vi "finishPulses.vi"(8 "error in (no error)":errorcluster, 11 "ScriptEvent in":refnum<class "ScriptEvent.lvclass">) -> (0 "error out":errorcluster, 2 "pulse finish":refnum<class "ScriptEvent.lvclass">, 3 "ScriptEvent out":refnum<class "ScriptEvent.lvclass">)   [LabVIEW 2011, in "Tools.lvlib" / "Scripting.lvlib" / "ScriptEvent.lvclass"]
uses:
  ScriptEvent.lvclass
  DatabaseHelpers/Database Objects/Channel/DigitalChannel/DigitalChannel.lvclass
  ScriptEvent.lvclass/ScriptEvent.ctl
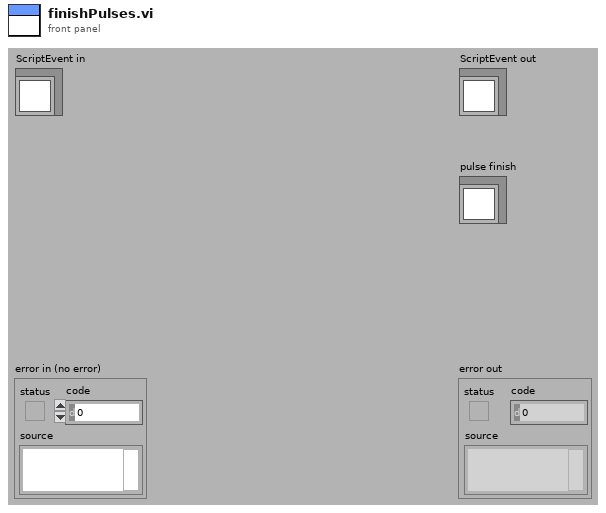
[diagram p1: front panel]
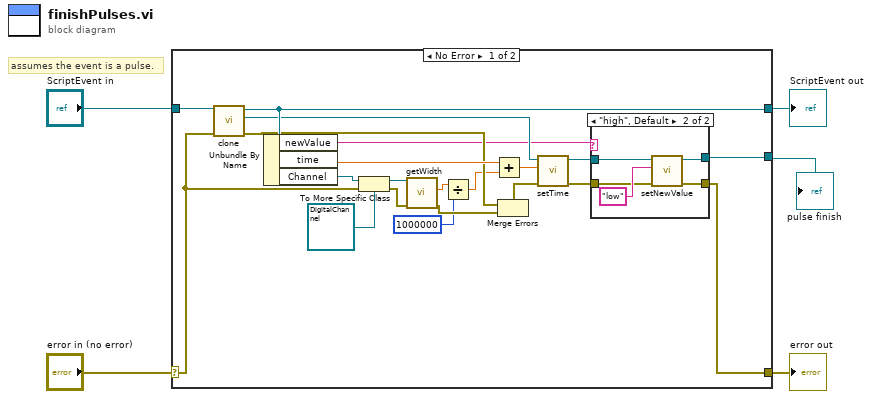
[diagram p0: block diagram]
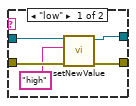
[diagram p2: hidden frame]
diagram:
  # "assumes the event is a pulse."
  n1 = case shown="No Error" "error in (no error)" {
    selector: "error in (no error)" -> [w21 w38]
    tunnel: [w10 w38] -> w4
    tunnel: [w25 w37] -> w2
    tunnel: "ScriptEvent in" -> [w26 w37]
    tunnel: [w9 _] -> w1
    frame No Error {
      n2 = call-dynamic "clone.vi"("error in (no error)"=w21, "ScriptEvent in"=w26) -> ("error out"=w18:errorcluster, "clone"=w20:refnum<class "ScriptEvent.lvclass">, "ScriptEvent out"=w25:refnum<class "ScriptEvent.lvclass">)  [unwired: 7 in]
      n3 = Unbundle By Name(w25) -> ("newValue"=w13:string, "time"=w24:dbl, "Channel"=w23:refnum<class "Channel.lvclass">)
      n4 = To More Specific Class(target class=refnum<class "DigitalChannel.lvclass"> refnum ("Tools.lvlib:DatabaseHelpers.lvlib:DigitalChannel.lvclass"), reference=w23, error in=w21) -> (specific class reference=w16:refnum<class "DigitalChannel.lvclass">, error out=w15:errorcluster)
      n5 = call "getWidth.vi"("error in (no error)"=w15, "DigitalChannel.lvclass in"=w16) -> ("error out"=w14:errorcluster, "width"=w8:dbl)  [unwired: 7 in, 1 out]
      n6 = Divide(x=w8, y=1000000) -> (x/y=w7:dbl)
      n7 = Add(x=w24, y=w7) -> (x+y=w19:dbl)
      n8 = Merge Errors(w18, w14) -> (w17:errorcluster)
      n9 = call "setTime.vi"("error in (no error)"=w17, "time"=w19, "ScriptEvent.lvclass in"=w20) -> ("error out"=w11:errorcluster, "ScriptEvent.lvclass out"=w12:refnum<class "ScriptEvent.lvclass">)  [unwired: 7 in]
      n10 = case shown="\"high\", Default" w13 {
        tunnel: w12 -> [w31 w36]
        tunnel: w11 -> [w30 w34]
        tunnel: [w29 w33] -> w10
        tunnel: [w28 w32] -> w9
        frame "low" {
          n11 = call "setNewValue.vi"("error in (no error)"=w30, "newValue"="high", "ScriptEvent.lvclass in"=w31) -> ("error out"=w29:errorcluster, "ScriptEvent.lvclass out"=w28:refnum<class "ScriptEvent.lvclass">)  [unwired: 7 in]
        }
        frame "high", Default {
          n12 = call "setNewValue.vi"("error in (no error)"=w34, "newValue"="low", "ScriptEvent.lvclass in"=w36) -> ("error out"=w33:errorcluster, "ScriptEvent.lvclass out"=w32:refnum<class "ScriptEvent.lvclass">)  [unwired: 7 in]
        }
      }
    }
    frame Error {
    }
  }
  "error out" <- w4
  "ScriptEvent out" <- w2
  "pulse finish" <- w1
